vi "Simple bead tracker.vi"() -> ()   [LabVIEW 2011]
uses:
  <vilib>/LapDog/Messaging.v2/MessageQueue/MessageQueue.lvclass
  Lib/Bead tracking settings.ctl
  <vilib>/LapDog/Messaging.v2/MessageQueue/EnqueueMessage(MsgName).vi
  Lib/COSYLib/COSYLib.lvlib
  <vilib>/vision/NI_Vision_Development_Module.lvlib
panel:
  in  "Pages":T1(tab)
  out "Template used":T2(plugin-control)
  in  "Pixel size (nm)":dbl=100.0 caption="Pixel size" min=0.01 max=1000.0 step=0.1 format="%#_g nm"
  in  "Subpixel accuracy":bool=TRUE
  in  "Minimum match score":sgl=250.0 min=0 step=100 format="%#_3g"
  out "First image in list":T2(plugin-control) caption="Please select your bead template in the image below, and click Next to continue:"
  in  "Refresh image directory":bool
  in  "Directory with images":path
  in  "Abort":bool
  out "Progress":u8(slide) caption="Please wait..." scale=0.0..100.0
  in  "Result tabs":enum32{"Plots", "Inspect tracking"}(tab)
  in  "D,t units":enum32{"um", "pix"}(radio) caption="Show graph in:"
  out "Match score graph":sgl[][](graph)
  out "Distance graph":dbl[](graph)
  in  "Index slider":u32(slide)=1 min=1 scale=1.0..9973.0
  out "Match info":T3(array[cluster]) {"Bounding Box"."y" format="%.2f"; "Bounding Box"."x" format="%.2f"; "Position"."y" format="%.2f"; "Position"."x" format="%.2f"; "Score" format="%.2f"; "Scale" format="%.2f"; "Angle" format="%.2f"}
  out "Result image":T2(plugin-control)
  in  "Export Results":bool
  in  "Next":bool
  # "Please run this VI to get started."
  # "Bead Tracking Settings"
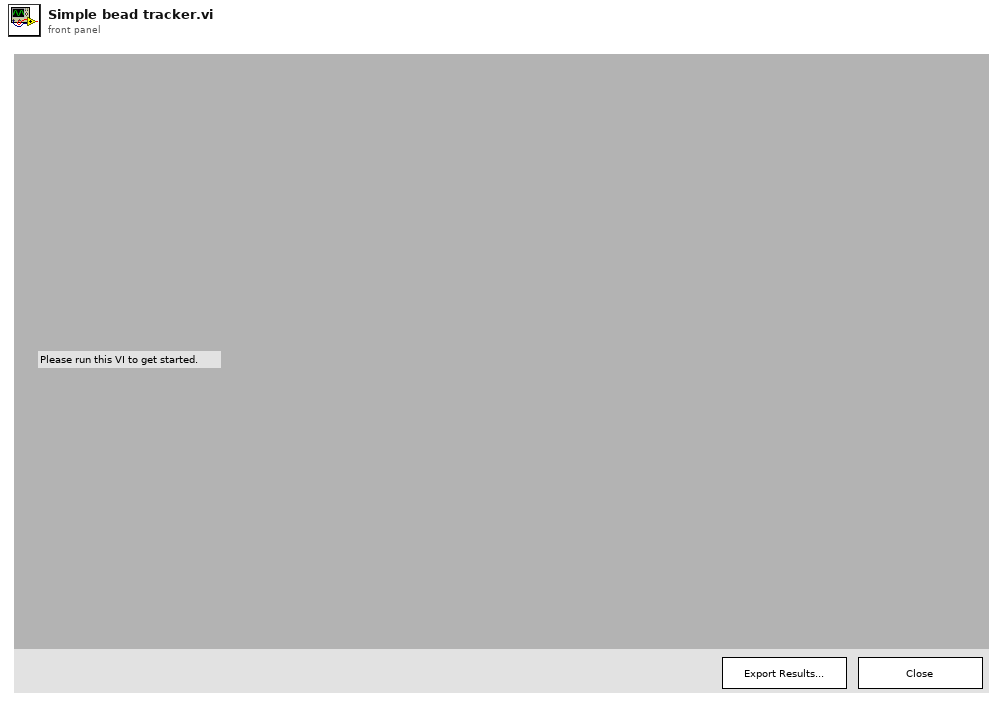
[diagram p1: front panel]
types:
  T1 = enum32{"Welcome", "Set up", "Processing", "Results"}
  T2 = typedef "IMAQ Image.ctl" = refnum<image>
  T3 = cluster{"Position":cluster{"x":sgl, "y":sgl}, "Angle":sgl, "Scale":sgl, "Score":sgl, "Bounding Box":cluster{"x":sgl, "y":sgl}[]}[]
  T4 = typedef "Image Type" = u32
  T5 = typedef "IMAQ Rectangle" = cluster{"Left":i32, "Top":i32, "Right":i32, "Bottom":i32, "Rotation":dbl}
  T6 = typedef "Bead tracking settings.ctl" = cluster{"Minimum match score":sgl, "Subpixel accuracy":bool, "Pixel calibration (nm/pix)":dbl}
  T7 = cluster{"Global Rectangle":i32[], "Contours":cluster{"Contour Type":u32, "ROI Type":u32, "Points":i32[]}[]}
  T8 = enum8{"Enabled", "Disabled", "Disabled and Grayed Out"}
  T9 = typedef "Worker result.ctl" = cluster{"Index":u32, "Distance (um)":dbl, "Raw matches":cluster{"Position":cluster{"x":sgl, "y":sgl}, "Angle":sgl, "Scale":sgl, "Score":sgl, "Bounding Box":cluster{"x":sgl, "y":sgl}[]}[], "File":path}
  T10 = cluster{"Position":cluster{"x":sgl, "y":sgl}, "Angle":sgl, "Scale":sgl, "Score":sgl, "Bounding Box":cluster{"x":sgl, "y":sgl}[]}
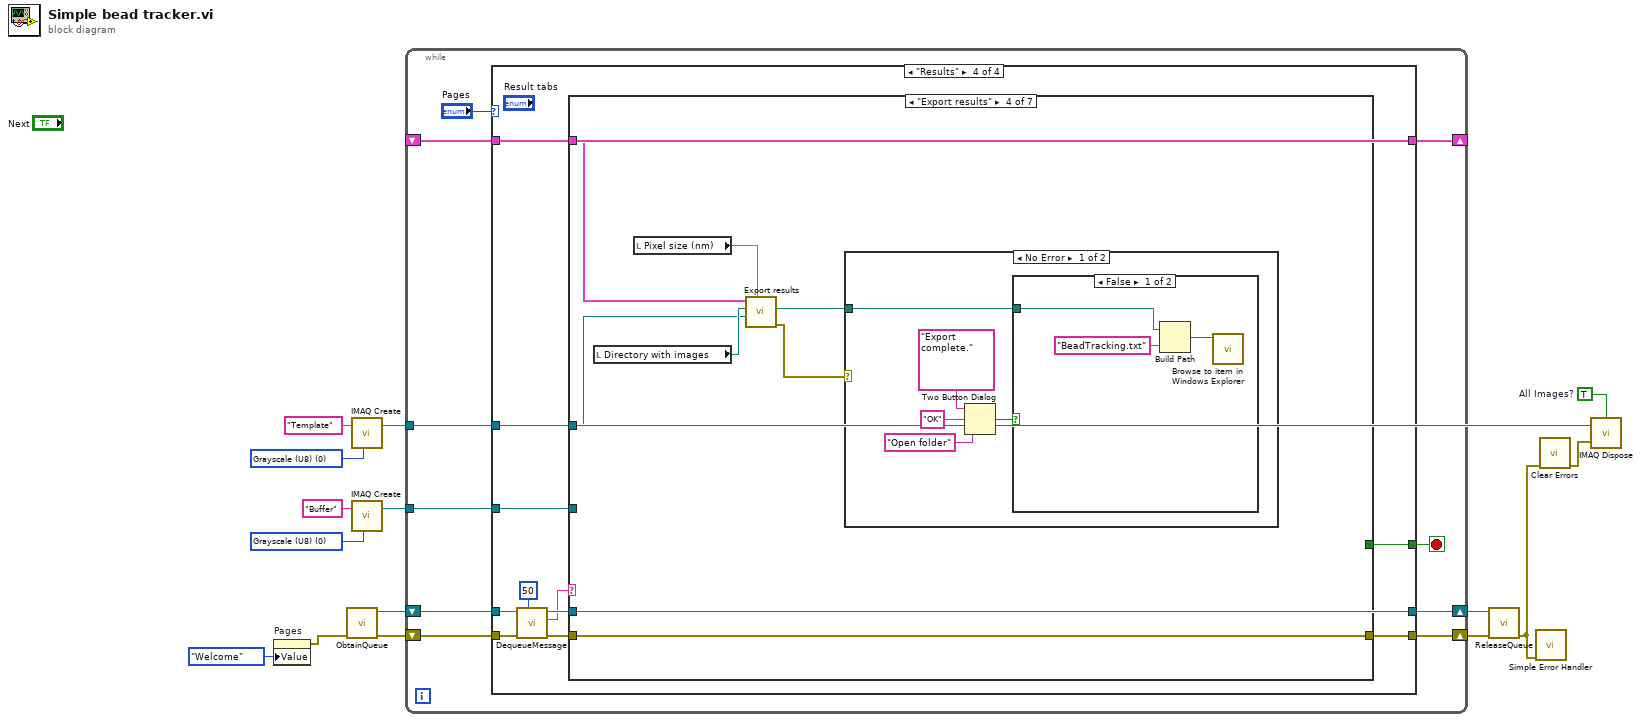
[diagram p0: block diagram]
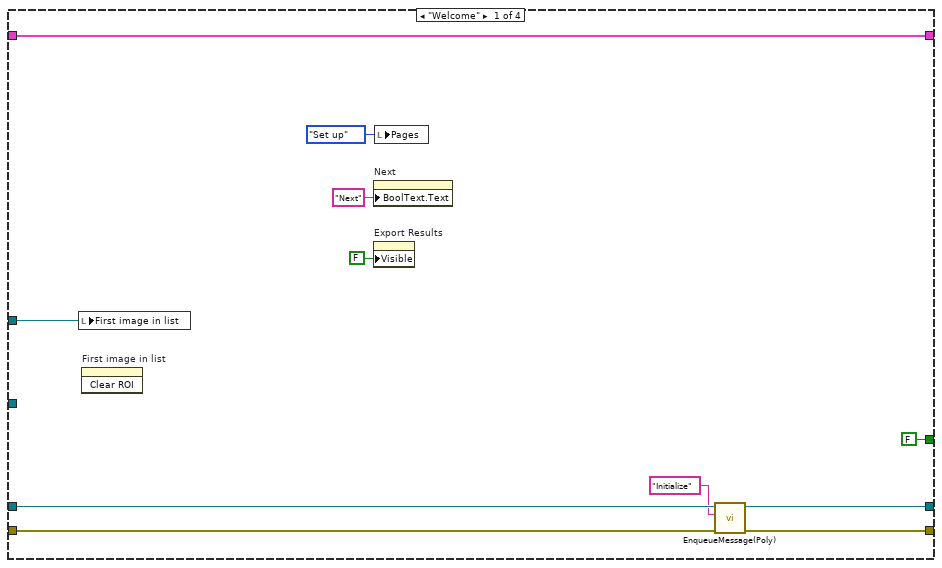
[diagram p2: hidden frame]
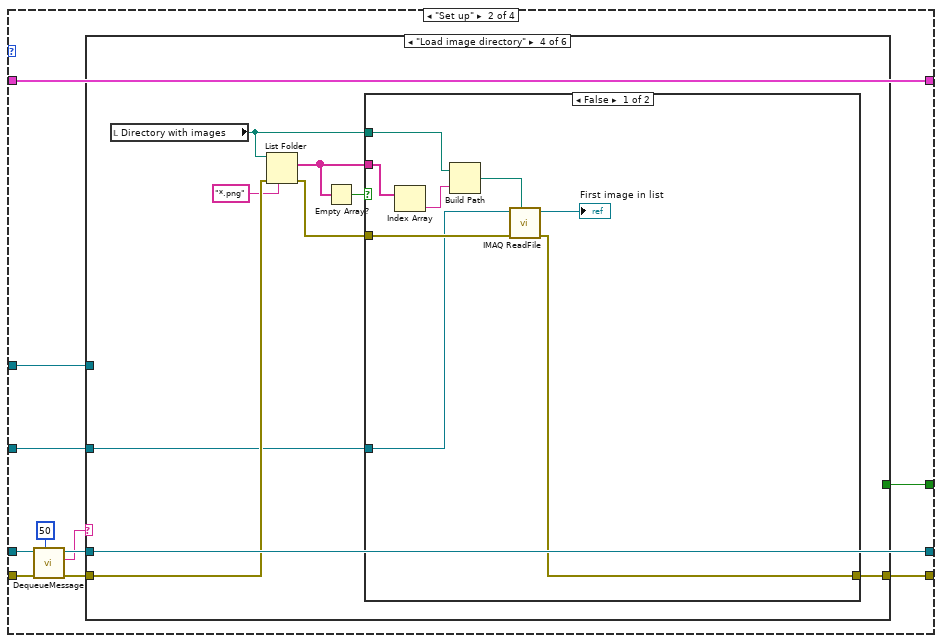
[diagram p3: hidden frame]
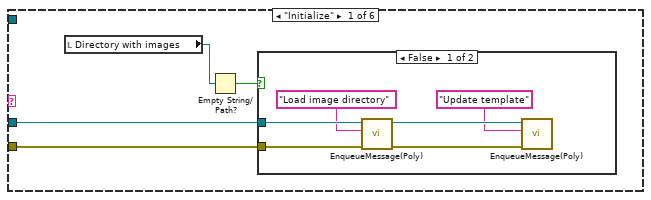
[diagram p4: hidden frame]
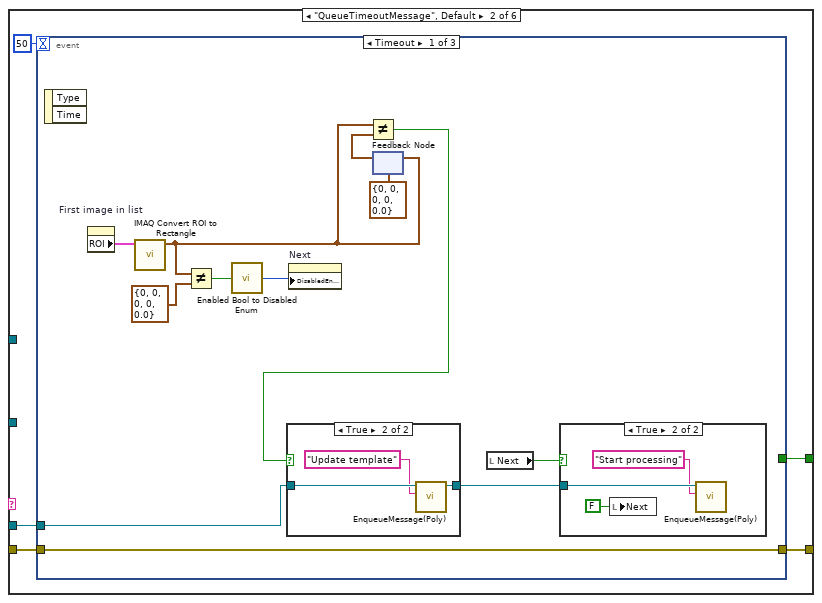
[diagram p6: hidden frame]
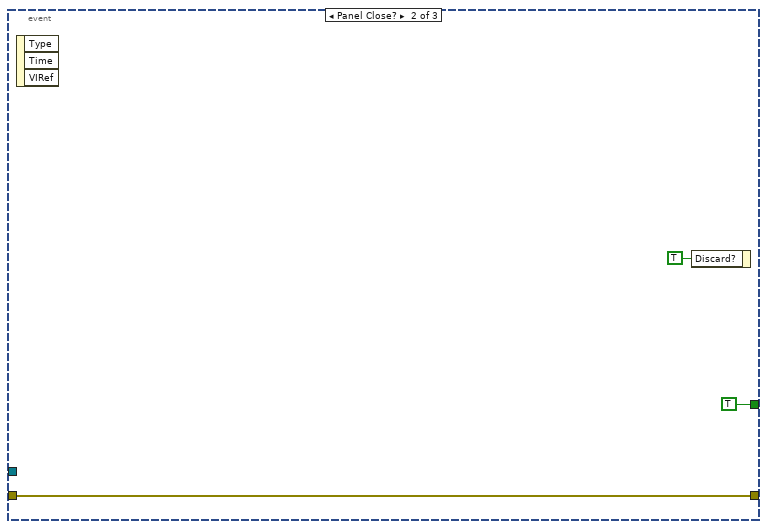
[diagram p9: hidden frame]
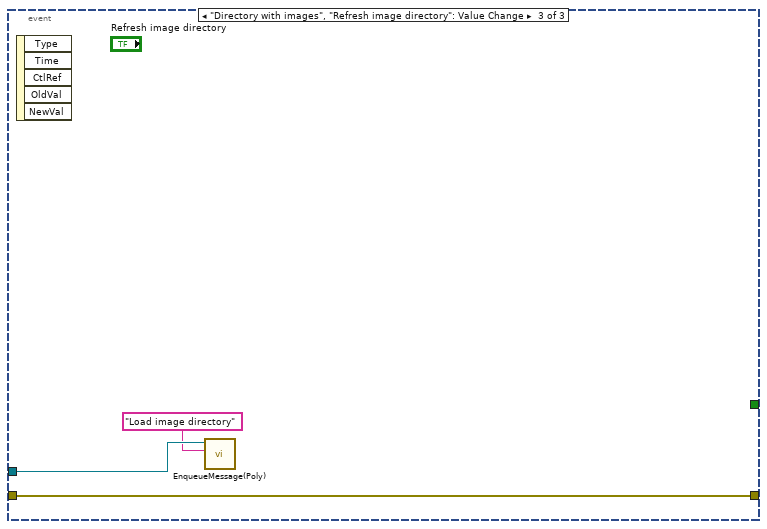
[diagram p10: hidden frame]
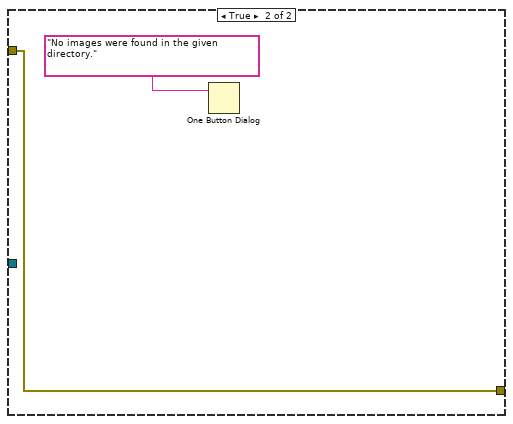
[diagram p12: hidden frame]
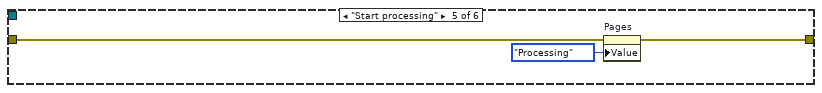
[diagram p13: hidden frame]
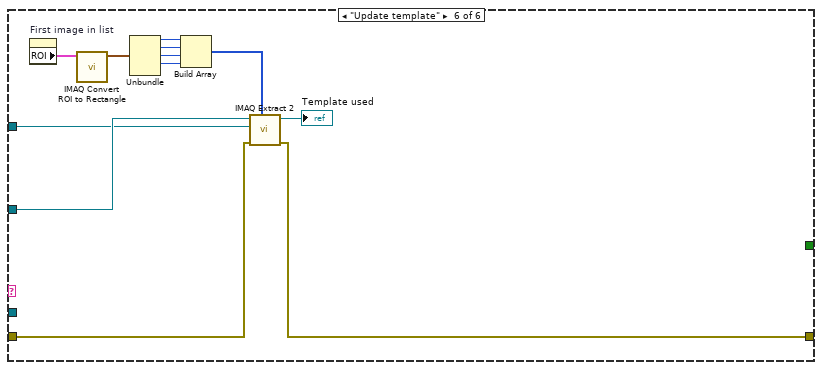
[diagram p14: hidden frame]
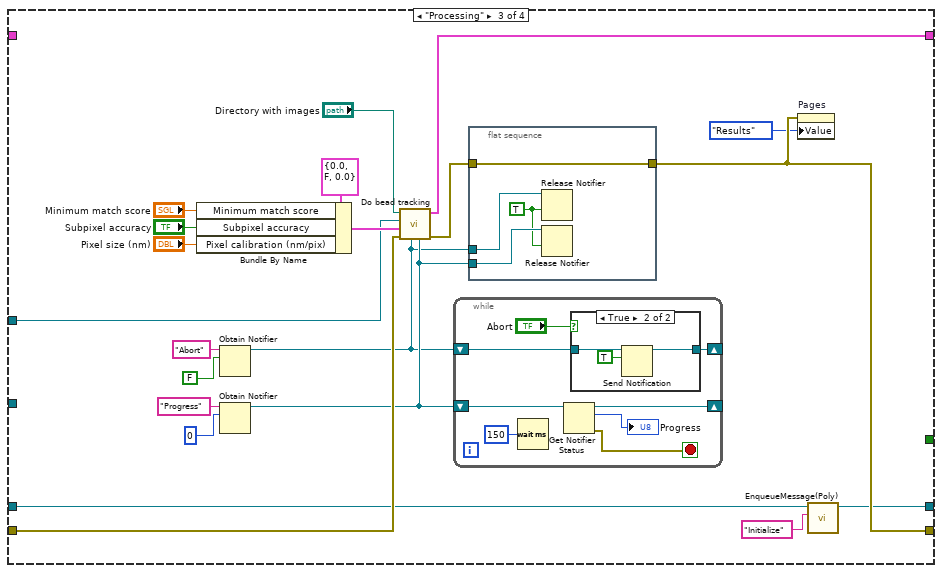
[diagram p15: hidden frame]
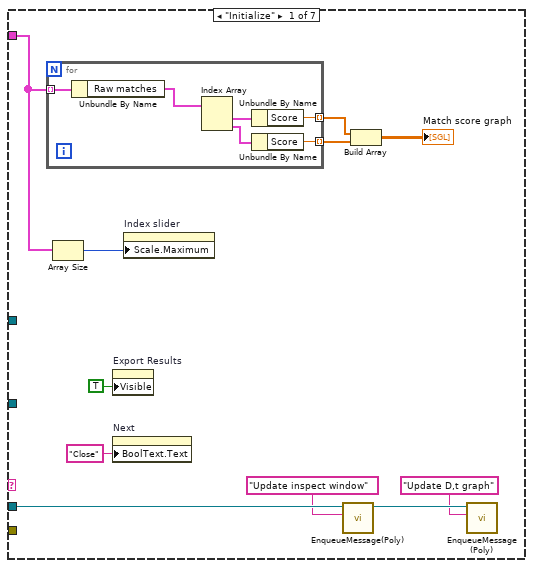
[diagram p17: hidden frame]
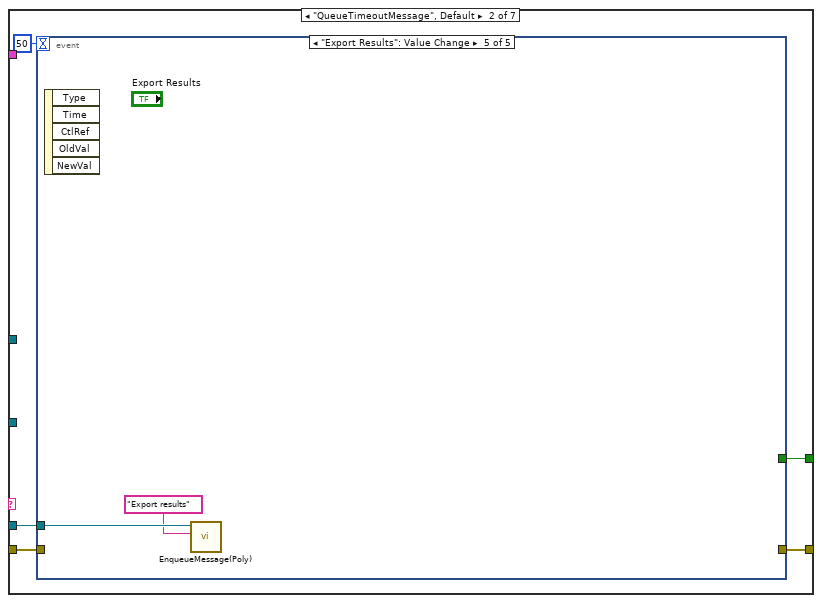
[diagram p18: hidden frame]
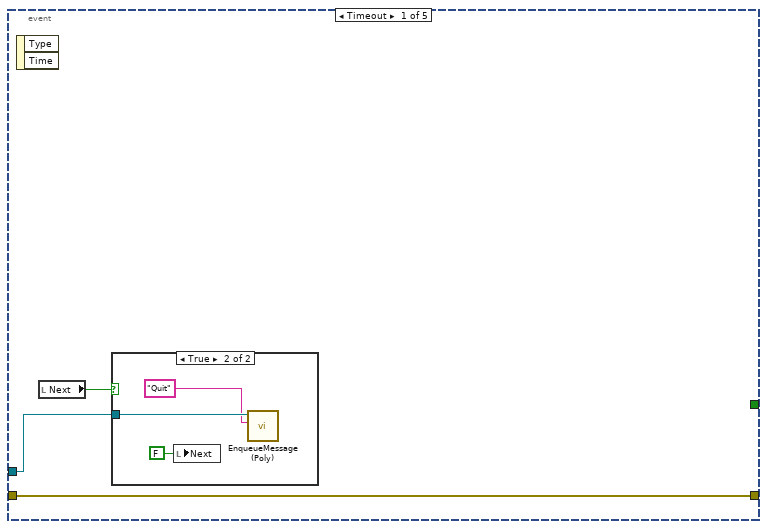
[diagram p19: hidden frame]
diagram:
  w2 = TRUE  # All Images?
  w6 = T4 0 items=["Grayscale (U8)", "Grayscale (I16)", "Grayscale (SGL)", "Complex (CSG)", "RGB (U32)", "HSL (U32)", "RGB (U64)", "Grayscale (U16)"] ("Image Type")
  w7 = T4 0 items=["Grayscale (U8)", "Grayscale (I16)", "Grayscale (SGL)", "Complex (CSG)", "RGB (U32)", "HSL (U32)", "RGB (U64)", "Grayscale (U16)"] ("Image Type")
  n1 = property on="Pages" class="TabCtl (strict)"("Value"=T1."Welcome" ("Pages")) -> (error out=w13:errorcluster)  [unwired: 2 in, 1 out]
  n2 = call <vilib>:"ObtainQueue.vi"("error in (no error)"=w13) -> ("error out"=w15:errorcluster, "MessageQueue out"=w10:refnum<class "MessageQueue.lvclass">)  [unwired: 8 in, 1 out]
  n3 = call "IMAQ Create"("Image Name"="Template", "Image Type"=w6) -> ("New Image"=w1:T2)  [unwired: 3 in, 1 out]
  n4 = call "IMAQ Create"("Image Name"="Buffer", "Image Type"=w7) -> ("New Image"=w4:T2)  [unwired: 3 in, 1 out]
  n5 = while {
    shift-right: [w21] -> w9
    shift-left: w10 -> [w22]
    shift-right: [w24] -> w14
    shift-left: w15 -> [w25]
    tunnel: w1 -> [w19]
    tunnel: w4 -> [w18]
    shift-right: [w17] -> _
    shift-left: _ -> [w16]
    stop <- w20 stop-if-true
    n6 = case shown="\"Results\"" "Pages" {
      tunnel: w22 -> [w32 w44 w139 w166]
      tunnel: [w31 w42 w124 w164] -> w21
      tunnel: w25 -> [w36 w47 w141 w169]
      tunnel: [w35 w45 w140 w167] -> w24
      tunnel: [FALSE w40 _ w162] -> w20
      tunnel: w19 -> [w33 w39 w132 w161]
      tunnel: w18 -> [_ w38 _ w160]
      tunnel: [w27 w37 w122 w159] -> w17
      tunnel: w16 -> [w27 w37 _ w159]
      frame "Welcome" {
        n7 = local write "First image in list"(w33) -> ()
        n8 = invoke on="First image in list" class="ImageControl" method="Clear ROI"() -> ()  [unwired: 3 in, 3 out]
        n9 = property on="Next" class="Bool (strict)"("BoolText.Text"="Next" ("Boolean Text.Text")) -> ()  [unwired: 2 in, 2 out]
        n10 = property on="Export Results" class="Bool"("Visible"=FALSE) -> ()  [unwired: 2 in, 2 out]
        n11 = local write "Pages"(enum32{"Welcome", "Set up", "Processing"}."Set up" ("Pages")) -> ()
        n12 = call-poly <vilib>:"EnqueueMessage(Poly).vi"("error in (no error)"=w36, "Message Name"="Initialize", "MessageQueue"=w32) -> ("error out"=w35:errorcluster, "MessageQueue out"=w31:refnum<class "MessageQueue.lvclass">)  [unwired: 6 in, 1 out]
      }
      frame "Set up" {
        n13 = call-dynamic "DequeueMessage.vi"("Timeout (-1 ms)"=50, "error in (no error)"=w47, "MessageQueue"=w44) -> ("error out"=w46:errorcluster, "Message Name"=w41:string, "MessageQueue out"=w42:refnum<class "MessageQueue.lvclass">)  [unwired: 4 in, 2 out]
        n14 = case shown="\"Load image directory\"" w41 {
          tunnel: w42 -> [w48 w59 _ _ _ _]
          tunnel: w46 -> [w51 w61 w88 w96 w107 w121]
          tunnel: [_ w62 w88 w94 w109 w111] -> w45
          tunnel: [_ w60 _ _ _ _] -> w40
          tunnel: w39 -> [_ _ _ _ _ w118]
          tunnel: w38 -> [_ _ _ w89 _ w119]
          frame "Initialize" {
            n15 = local read "Directory with images"() -> (w50:path)
            n16 = Empty String/Path?(string/path=w50) -> (empty?=w49:bool)
            n17 = case shown="False" w49 {
              tunnel: w48 -> [w55 _]
              tunnel: w51 -> [w56 _]
              frame False {
                n18 = call-poly <vilib>:"EnqueueMessage(Poly).vi"("error in (no error)"=w56, "Message Name"="Load image directory", "MessageQueue"=w55) -> ("error out"=w52:errorcluster, "MessageQueue out"=w57:refnum<class "MessageQueue.lvclass">)  [unwired: 6 in, 1 out]
                n19 = call-poly <vilib>:"EnqueueMessage(Poly).vi"("error in (no error)"=w52, "Message Name"="Update template", "MessageQueue"=w57) -> ()  [unwired: 6 in, 3 out]
              }
              frame True {
              }
            }
          }
          frame "QueueTimeoutMessage", Default {
            n20 = event shown="[0] Timeout" {
              selector: _ -> [_ _ _]
              dyn-events: _ -> [_ _ _]
              timeout: 50 -> [_ _ _]
              tunnel: [w74 w84 w87] -> w62
              tunnel: w61 -> [w74 w84 w87]
              tunnel: [_ TRUE _] -> w60
              tunnel: w59 -> [w64 _ w86]
              event Timeout {
                n21 = event-data() -> ()  [unwired: 1 in, 2 out]
                n22 = property on="First image in list" class="ImageControl"() -> ("ROI"=w73:T7)  [unwired: 2 in, 2 out]
                n23 = call "IMAQ Convert ROI to Rectangle"("ROI Descriptor"=w73) -> ("Rectangle"=w67:T5)  [unwired: 8 in, 1 out]
                n24 = Not Equal?(x=w67, y=T5 {"Left"=0, "Top"=0, "Right"=0, "Bottom"=0, "Rotation"=0.0} ("Rectangle")) -> (x != y?=w71:bool)
                n25 = call "Enabled Bool to Disabled Enum.vi"("Enabled?"=w71) -> ("Disabled"=w70:T8)
                n26 = property on="Next" class="Bool (strict)"("DisabledEnum"=w70) -> ()  [unwired: 2 in, 2 out]
                n27 = feedback-in #1(w67) -> ()
                n28 = feedback #1(T5 {"Left"=0, "Top"=0, "Right"=0, "Bottom"=0, "Rotation"=0.0} ("Rectangle")) -> (w68:T5)
                n29 = Not Equal?(x=w67, y=w68) -> (x != y?=w66:bool)
                n30 = case shown="True" w66 {
                  tunnel: w64 -> [w75 w78]
                  tunnel: [w75 w76] -> w63
                  frame False {
                  }
                  frame True {
                    n31 = call-poly <vilib>:"EnqueueMessage(Poly).vi"("Message Name"="Update template", "MessageQueue"=w78) -> ("MessageQueue out"=w76:refnum<class "MessageQueue.lvclass">)  [unwired: 7 in, 2 out]
                  }
                }
                n32 = local read "Next"() -> (w69:bool)
                n33 = case shown="True" w69 {
                  tunnel: w63 -> [_ w81]
                  frame False {
                  }
                  frame True {
                    n34 = local write "Next"(FALSE ("Next")) -> ()
                    n35 = call-poly <vilib>:"EnqueueMessage(Poly).vi"("Message Name"="Start processing", "MessageQueue"=w81) -> ()  [unwired: 7 in, 3 out]
                  }
                }
              }
              event Panel Close? {
                n36 = event-data() -> ()  [unwired: 1 in, 3 out]
                n37 = event-data("Discard?"=TRUE) -> ()  [unwired: 1 in, 1 out]
              }
              event "Directory with images", "Refresh image directory": Value Change {
                n38 = event-data() -> ()  [unwired: 1 in, 5 out]
                n39 = call-poly <vilib>:"EnqueueMessage(Poly).vi"("Message Name"="Load image directory", "MessageQueue"=w86) -> ()  [unwired: 7 in, 3 out]
              }
            }
          }
          frame "------------------------------------" {
          }
          frame "Load image directory" {
            n40 = local read "Directory with images"() -> (w90:path)
            n41 = List Folder(path=w90, pattern="*.png", error in=w96) -> (filenames=w91:string[], error out=w95:errorcluster)  [unwired: 1 in, 2 out]
            n42 = Empty Array?(array=w91) -> (empty?=w92:bool)
            n43 = case shown="False" w92 {
              tunnel: w91 -> [w102 _]
              tunnel: w90 -> [w101 _]
              tunnel: w95 -> [w104 w106]
              tunnel: [w103 w106] -> w94
              tunnel: w89 -> [w97 _]
              frame False {
                n44 = Index Array(array=w102) -> (element=w100:string)  [unwired: 1 in]
                n45 = Build Path(base path=w101, name or relative path=w100) -> (appended path=w99:path)
                n46 = call "IMAQ ReadFile"("File Path"=w99, "error in (no error)"=w104, "Image"=w97) -> ("error out"=w103:errorcluster, "Image Out"=→"First image in list":T2)  [unwired: 4 in, 3 out]
              }
              frame True {
                n47 = One Button Dialog(message="No images were found in the given directory.") -> ()  [unwired: 1 in, 1 out]
              }
            }
          }
          frame "Start processing" {
            n48 = property on="Pages" class="TabCtl (strict)"(error in=w107, "Value"=T1."Processing" ("Pages")) -> (error out=w109:errorcluster)  [unwired: 1 in, 1 out]
          }
          frame "Update template" {
            n49 = property on="First image in list" class="ImageControl"() -> ("ROI"=w120:T7)  [unwired: 2 in, 2 out]
            n50 = call "IMAQ Convert ROI to Rectangle"("ROI Descriptor"=w120) -> ("Rectangle"=w117:T5)  [unwired: 8 in, 1 out]
            n51 = Unbundle(w117) -> ("Left"=w116:i32, "Top"=w115:i32, "Right"=w114:i32, "Bottom"=w113:i32)  [unwired: 1 out]
            n52 = Build Array(w116, w115, w114, w113) -> (w112:i32[])
            n53 = call "IMAQ Extract 2"("Optional Rectangle"=w112, "error in (no error)"=w121, "Image Dst"=w118, "Image Src"=w119) -> ("error out"=w111:errorcluster, "Image Dst Out"=→"Template used":T2)  [unwired: 6 in]
          }
        }
      }
      frame "Processing" {
        n54 = Bundle By Name(cluster=T6 {"Minimum match score"=0.0, "Subpixel accuracy"=FALSE, "Pixel calibration (nm/pix)"=0.0} ("Bead tracking settings"), "Minimum match score"="Minimum match score", "Subpixel accuracy"="Subpixel accuracy", "Pixel calibration (nm/pix)"="Pixel size (nm)") -> (w134:T6)
        n55 = Obtain Notifier(name (unnamed)="Abort", notification data type=FALSE) -> (notifier out=w126:refnum<notifier>)  [unwired: 2 in, 2 out]
        n56 = Obtain Notifier(name (unnamed)="Progress", notification data type=u8 0) -> (notifier out=w127:refnum<notifier>)  [unwired: 2 in, 2 out]
        n57 = call "Do bead tracking.vi"("Progress notf"=w127, "Abort notf"=w126, "error in (no error)"=w141, "Bead tracking settings"=w134, "Template"=w132, "Directory"="Directory with images") -> ("error out"=w142:errorcluster, "Results"=w122:T9[])  [unwired: 4 in]
        n58 = while {
          shift-right: [w152] -> _
          shift-left: w126 -> [w151]
          shift-right: [w149] -> _
          shift-left: w127 -> [w150]
          stop <- w154 stop-if-true
          n59 = Wait (ms)(milliseconds to wait=u32 150) -> ()  [unwired: 1 out]
          n60 = Get Notifier Status(notifier=w150) -> (notifier out=w149:refnum<notifier>, current notification=→"Progress":u8, error out=w154:errorcluster)  [unwired: 1 in, 2 out]
          n61 = case shown="True" "Abort" {
            tunnel: [w155 w157] -> w152
            tunnel: w151 -> [w155 w158]
            frame False {
            }
            frame True {
              n62 = Send Notification(notification=TRUE, notifier=w158) -> (notifier out=w157:refnum<notifier>)  [unwired: 1 in, 1 out]
            }
          }
        }
        n63 = flat-sequence {
          tunnel: w127 -> [w144]
          tunnel: w126 -> [w145]
          tunnel: w142 -> [w146]
          tunnel: [w146] -> w140
          frame #0 {
            w143 = TRUE ("force destroy? (F)")
            n64 = Release Notifier(notifier=w145, force destroy? (F)=w143) -> ()  [unwired: 1 in, 3 out]
            n65 = Release Notifier(notifier=w144, force destroy? (F)=w143) -> ()  [unwired: 1 in, 3 out]
          }
        }
        n66 = property on="Pages" class="TabCtl (strict)"(error in=w140, "Value"=T1."Results" ("Pages")) -> ()  [unwired: 1 in, 2 out]
        n67 = call-poly <vilib>:"EnqueueMessage(Poly).vi"("Message Name"="Initialize", "MessageQueue"=w139) -> ("MessageQueue out"=w124:refnum<class "MessageQueue.lvclass">)  [unwired: 7 in, 2 out]
      }
      frame "Results" {
        n68 = call-dynamic "DequeueMessage.vi"("Timeout (-1 ms)"=50, "error in (no error)"=w169, "MessageQueue"=w166) -> ("error out"=w168:errorcluster, "Message Name"=w163:string, "MessageQueue out"=w164:refnum<class "MessageQueue.lvclass">)  [unwired: 4 in, 2 out]
        n69 = case shown="\"Export results\"" w163 {
          tunnel: w164 -> [w173 w188 _ _ _ _ _]
          tunnel: w168 -> [_ w190 w208 w215 w234 w240 w252]
          tunnel: [_ w191 w208 w215 w234 w240 w252] -> w167
          tunnel: [_ w189 _ _ _ _ TRUE] -> w162
          tunnel: w161 -> [_ _ _ w213 _ _ _]
          tunnel: w160 -> [_ _ _ _ w229 _ _]
          tunnel: w159 -> [w175 _ _ w212 w232 w239 _]
          frame "Initialize" {
            n70 = for {
              tunnel: w175 -> [w186] mode=indexing
              tunnel: [w182] -> w178 mode=indexing
              tunnel: [w181] -> w177 mode=indexing
              n71 = Unbundle By Name(w186) -> ("Raw matches"=w185:T3)
              n72 = Index Array(array=w185) -> (element #1=w184:T10, element #2=w183:T10)  [unwired: 2 in]
              n73 = Unbundle By Name(w184) -> ("Score"=w182:sgl)
              n74 = Unbundle By Name(w183) -> ("Score"=w181:sgl)
            }
            n75 = Array Size(array=w175) -> (size(s)=w174:i32)
            n76 = property on="Export Results" class="Bool"("Visible"=TRUE) -> ()  [unwired: 2 in, 2 out]
            n77 = property on="Next" class="Bool (strict)"("BoolText.Text"="Close" ("Boolean Text.Text")) -> ()  [unwired: 2 in, 2 out]
            n78 = property on="Index slider" class="Slide (strict)"("Scale.Maximum"=w174) -> ()  [unwired: 2 in, 2 out]
            n79 = call-poly <vilib>:"EnqueueMessage(Poly).vi"("Message Name"="Update inspect window", "MessageQueue"=w173) -> ("MessageQueue out"=w180:refnum<class "MessageQueue.lvclass">)  [unwired: 7 in, 2 out]
            n80 = Build Array(w178, w177) -> (→"Match score graph":sgl[][])
            n81 = call-poly <vilib>:"EnqueueMessage(Poly).vi"("Message Name"="Update D,t graph", "MessageQueue"=w180) -> ()  [unwired: 7 in, 3 out]
          }
          frame "QueueTimeoutMessage", Default {
            n82 = event shown="[4] \"Export Results\": Value Change" {
              selector: _ -> [_ _ _ _ _]
              dyn-events: _ -> [_ _ _ _ _]
              timeout: 50 -> [_ _ _ _ _]
              tunnel: [w194 w200 w203 _ _] -> w191
              tunnel: w190 -> [w194 w200 w203 _ _]
              tunnel: [_ _ TRUE _ _] -> w189
              tunnel: w188 -> [w192 w199 _ w205 w207]
              event Timeout {
                n83 = event-data() -> ()  [unwired: 1 in, 2 out]
                n84 = local read "Next"() -> (w193:bool)
                n85 = case shown="True" w193 {
                  tunnel: w192 -> [_ w197]
                  frame False {
                  }
                  frame True {
                    n86 = local write "Next"(FALSE ("Next")) -> ()
                    n87 = call-poly <vilib>:"EnqueueMessage(Poly).vi"("Message Name"="Quit", "MessageQueue"=w197) -> ()  [unwired: 7 in, 3 out]
                  }
                }
              }
              event "Index slider": Value Change {
                n88 = event-data() -> ()  [unwired: 1 in, 5 out]
                n89 = call-poly <vilib>:"EnqueueMessage(Poly).vi"("Message Name"="Update inspect window", "MessageQueue"=w199) -> ()  [unwired: 7 in, 3 out]
              }
              event Panel Close? {
                n90 = event-data() -> ()  [unwired: 1 in, 3 out]
                n91 = event-data("Discard?"=TRUE) -> ()  [unwired: 1 in, 1 out]
              }
              event "D,t units": Value Change {
                n92 = event-data() -> ()  [unwired: 1 in, 5 out]
                n93 = call-poly <vilib>:"EnqueueMessage(Poly).vi"("Message Name"="Update D,t graph", "MessageQueue"=w205) -> ()  [unwired: 7 in, 3 out]
              }
              event "Export Results": Value Change {
                n94 = event-data() -> ()  [unwired: 1 in, 5 out]
                n95 = call-poly <vilib>:"EnqueueMessage(Poly).vi"("Message Name"="Export results", "MessageQueue"=w207) -> ()  [unwired: 7 in, 3 out]
              }
            }
          }
          frame "------------------------------------" {
          }
          frame "Export results" {
            n96 = local read "Directory with images"() -> (w214:path)
            n97 = local read "Pixel size (nm)"() -> (w211:dbl)
            n98 = call "Export results.vi"("Pixel size (nm)"=w211, "Template Image"=w213, "Directory with images"=w214, "Results"=w212) -> ("error out"=w210:errorcluster, "Created results dir"=w209:path)  [unwired: 6 in]
            n99 = case shown="No Error" w210 {
              selector: w210 -> [_ w224]
              tunnel: w209 -> [w216 _]
              frame No Error {
                n100 = Two Button Dialog(message="Export complete.", 1:"Open folder" ("F button name (\"Cancel\")"), 2:"OK" ("T button name (\"OK\")")) -> (T button?=w219:bool)
                n101 = case shown="False" w219 {
                  tunnel: w216 -> [w223 _]
                  frame False {
                    n102 = Build Path(base path=w223, name or relative path="BeadTracking.txt") -> (appended path=w222:path)
                    n103 = call "Browse to item in Windows Explorer.vi"("File"=w222) -> ()  [unwired: 10 in, 1 out]
                  }
                  frame True {
                  }
                }
              }
              frame Error {
                n104 = call <vilib>:"Simple Error Handler.vi"("error in (no error)"=w224) -> ()  [unwired: 4 in, 5 out]
              }
            }
          }
          frame "Update inspect window" {
            n105 = Decrement(x="Index slider") -> (x-1=w231:u32)
            n106 = Index Array(array=w232, index=w231) -> (element=w228:T9)
            n107 = Unbundle By Name(w228) -> ("Raw matches"=w225:T3)
            "Match info" <- w225
            n108 = Unbundle By Name(w228) -> ("File"=w230:path)
            n109 = call "IMAQ ReadFile"("File Path"=w230, "Image"=w229) -> ("Image Out"=w226:T2)  [unwired: 5 in, 4 out]
            n110 = call "Draw matches in inspection image.vi"("Raw matches"=w225, "Image in"=w226) -> ("Image out"=→"Result image":T2)  [unwired: 9 in]
          }
          frame "Update D,t graph" {
            n111 = for {
              tunnel: w239 -> [w250] mode=indexing
              tunnel: [w249] -> w237 mode=indexing
              n112 = Unbundle By Name(w250) -> ("Distance (um)"=w249:dbl)
            }
            n113 = case shown="\"pix\"" "D,t units" {
              tunnel: w237 -> [w242 w248]
              tunnel: [w242 w244] -> w236
              tunnel: ["Distance (um)" "Distance (pix)"] -> w235
              frame "um" {
              }
              frame "pix" {
                n114 = local read "Pixel size (nm)"() -> (w245:dbl)
                n115 = Multiply(x=w248, y=1000.0) -> (x*y=w246:dbl[])
                n116 = Divide(x=w246, y=w245) -> (x/y=w244:dbl[])
              }
            }
            "Distance graph" <- w236
            n117 = property on="Distance graph" class="WFGraph (strict)"("YScale.NameLbl.Text"=w235) -> ()  [unwired: 2 in, 2 out]
          }
          frame "Quit" {
          }
        }
      }
    }
  }
  n118 = call-dynamic "ReleaseQueue.vi"("error in (no error)"=w14, "MessageQueue in"=w9) -> ("error out"=w11:errorcluster)  [unwired: 7 in, 2 out]
  n119 = call <vilib>:"Simple Error Handler.vi"("error in (no error)"=w11) -> ()  [unwired: 4 in, 5 out]
  n120 = call <vilib>:"Clear Errors.vi"("error in (no error)"=w11) -> ("error out"=w12:errorcluster)  [unwired: 6 in]
  n121 = call "IMAQ Dispose"("All Images? (No)"=w2, "Image"=w1, "error in (no error)"=w12) -> ()  [unwired: 3 in, 1 out]
